vi "ClassNode_GetMethodAtMouse.vi"(5 "MousePos":T1 {"y" format="%.2f"; "x" format="%.2f"}, 6 "error in":errorcluster, 7 "botHeight":dbl, 8 "bounds":T2 {"height" format="%.2f"; "width" format="%.2f"; "y" format="%.2f"; "x" format="%.2f"}, 9 "methods":refnum<class "MultiLineString.lvclass">) -> (0 "error out":errorcluster, 1 "MethodSelected":bool, 2 "NoMmethodsExists":bool, 3 "MEthodName":string)   [LabVIEW 2016, in "ClassNode.lvclass"]
uses:
  <resource>/Framework/Providers/Open_GDS/UML/ClassNode_class/ClassNode.lvclass
  <resource>/Framework/Providers/Open_GDS/UML/General/Rectangle/Rectangle Rectangle2D.ctl
  <resource>/Framework/Providers/Open_GDS/UML/General/Point/Point Point2D.ctl
  <resource>/Framework/Providers/Open_GDS/UML/MultiLineString_class/MultiLineString.lvclass
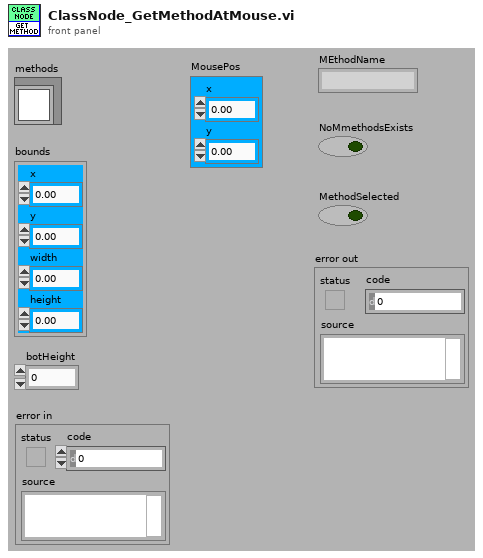
[diagram p1: front panel]
types:
  T1 = typedef "Point Point2D.ctl" = cluster{"x":dbl, "y":dbl}
  T2 = typedef "Rectangle Rectangle2D.ctl" = cluster{"x":dbl, "y":dbl, "width":dbl, "height":dbl}
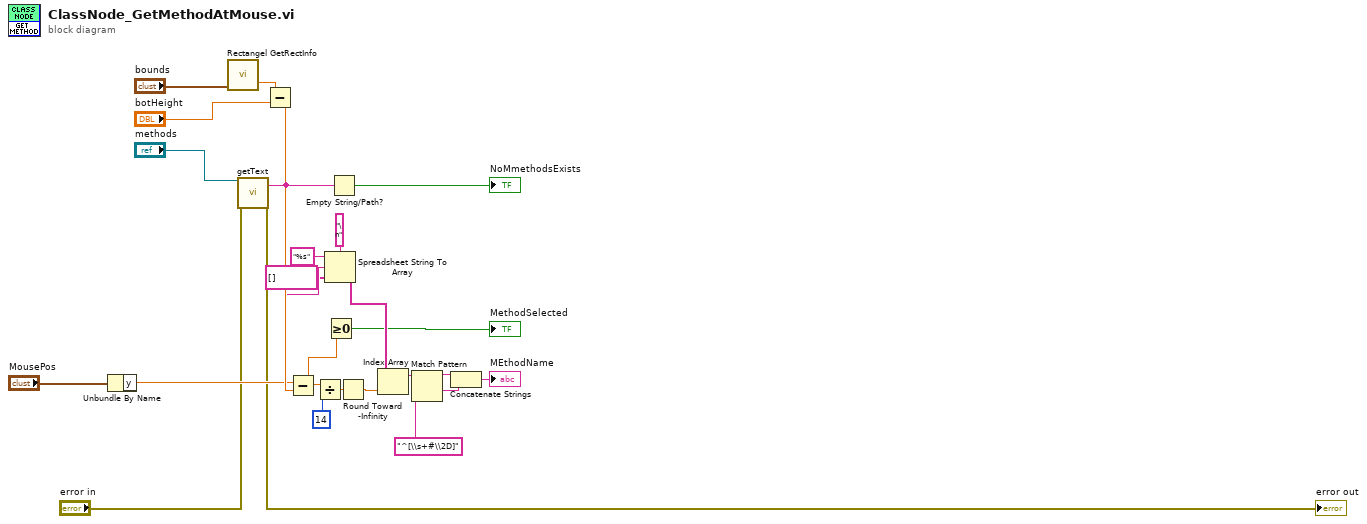
[diagram p0: block diagram]
diagram:
  n1 = Unbundle By Name("MousePos") -> ("y"=w13:dbl)
  n2 = call <resource>:"Rectangel GetRectInfo.vi"("bounds"="bounds") -> ("maxY"=w9:dbl)  [unwired: 1 in, 17 out]
  n3 = call-dynamic "getText.vi"("reference"="methods", "error in (no error)"="error in") -> ("text"=w11:string, "error out"=→"error out":errorcluster)  [unwired: 16 out]
  n4 = Subtract(x=w9, y="botHeight") -> (x-y=w14:dbl)
  n5 = Subtract(x=w13, y=w14) -> (x-y=w19:dbl)
  n6 = Divide(x=w19, y=14) -> (x/y=w17:dbl)
  n7 = Spreadsheet String To Array(delimiter (Tab)="\n", format string="%s", spreadsheet string=w11, array type (2D Dbl)=string[] []) -> (array=w20:string[])
  n8 = Greater Or Equal To 0?(x=w19) -> (x >= 0?=→"MethodSelected":bool)
  n9 = Empty String/Path?(string/path=w11) -> (empty?=→"NoMmethodsExists":bool)
  n10 = Round Toward -Infinity(1:w17) -> (0:w16:dbl)
  n11 = Index Array(array=w20, index=w16) -> (element=w24:string)
  n12 = Match Pattern(string=w24, regular expression="^[\\s+#\\2D]") -> (before substring=w22:string, after substring=w21:string)  [unwired: 3 out]
  n13 = Concatenate Strings(w22, w21) -> (→"MEthodName":string)
